vi "正常至16进制显示.vi"(11 "字符串_正常":string) -> (2 "字符串_16进制":string)   [LabVIEW 2010]
panel:
  # "用户串口写数据"
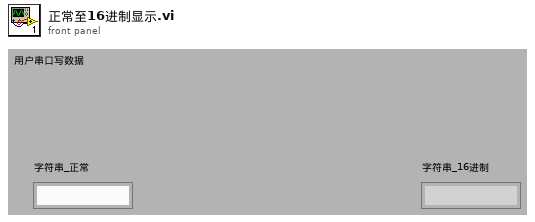
[diagram p1: front panel]
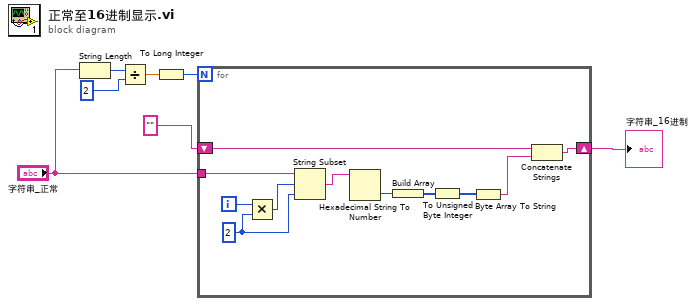
[diagram p0: block diagram]
diagram:
  n1 = String Length(string="字符串_正常") -> (length=w7:i32)
  n2 = Divide(x=w7, y=2) -> (x/y=w4:dbl)
  n3 = To Long Integer(number=w4) -> (32bit integer=w5:i32)
  n4 = for {
    N: w5 -> [_]
    tunnel: "字符串_正常" -> [w17]
    shift-right: [w8] -> w1
    shift-left: "" -> [w10]
    i -> [w18]
    w15 = 2 ("y")
    n5 = Multiply(x=w18, y=w15) -> (x*y=w16:i32)
    n6 = String Subset(string=w17, offset (0)=w16, length (rest)=w15) -> (substring=w14:string)
    n7 = Hexadecimal String To Number(string=w14) -> (number=w13:u32)  [unwired: 2 in, 1 out]
    n8 = Build Array(w13) -> (w12:u32[])
    n9 = To Unsigned Byte Integer(number=w12) -> (unsigned 8bit integer=w11:u8[])
    n10 = Byte Array To String(unsigned byte array=w11) -> (string=w9:string)
    n11 = Concatenate Strings(w10, w9) -> (w8:string)
  }
  "字符串_16进制" <- w1
